vi "sub_Test_main.vi"(8 "error in":errorcluster) -> (0 "error out":errorcluster)   [LabVIEW 2019]
uses:
  _ctrl/create-rw-close.ctl
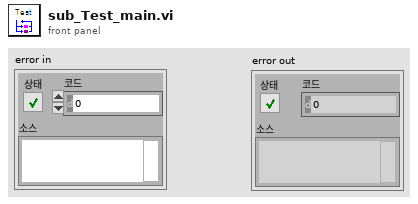
[diagram p1: front panel]
types:
  T1 = typedef "create-rw-close.ctl" = enum16{"create", "write", "read", "delete", "close"}
  T2 = typedef "fgv_Main_q.ctl" = enum16{"init", "wait", "R", "RC", "RC_M", "B1", "B2", "B3", "exit"}
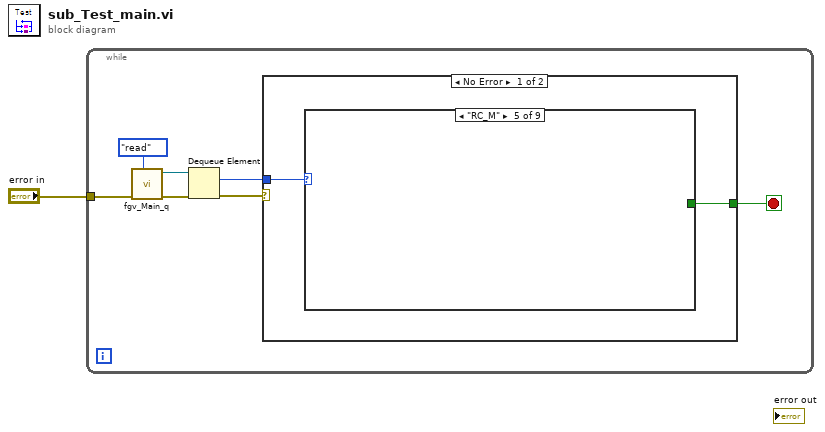
[diagram p0: block diagram]
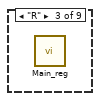
[diagram p4: hidden frame]
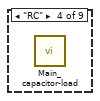
[diagram p5: hidden frame]
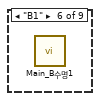
[diagram p6: hidden frame]
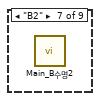
[diagram p7: hidden frame]
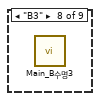
[diagram p8: hidden frame]
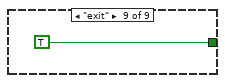
[diagram p9: hidden frame]
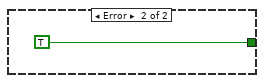
[diagram p10: hidden frame]
diagram:
  n1 = while {
    tunnel: "error in" -> [w2]
    stop <- w8 stop-if-true
    n2 = call "fgv_Main_q.vi"("cmd"=create-rw-close."read", "error in"=w2) -> ("error out"=w5:errorcluster, "queue out"=w6:refnum<queue>)  [unwired: 8 in]
    n3 = Dequeue Element(queue=w6, error in (no error)=w5) -> (element=w4:T2, error out=w3:errorcluster)  [unwired: 1 in, 2 out]
    n4 = case shown="No Error" w3 {
      tunnel: [w9 TRUE] -> w8
      tunnel: w4 -> [w10 _]
      frame No Error {
        n5 = case shown="\"RC_M\"" w10 {
          tunnel: [_ _ _ _ _ _ _ _ TRUE] -> w9
          frame "init", Default {
          }
          frame "wait" {
          }
          frame "R" {
            n6 = call "Main_reg.vi"() -> ()  [unwired: 12 in]
          }
          frame "RC" {
            n7 = call "Main_capacitor-load.vi"() -> ()  [unwired: 11 in, 1 out]
          }
          frame "RC_M" {
          }
          frame "B1" {
            n8 = call "Main_B수명1.vi"() -> ()  [unwired: 11 in, 1 out]
          }
          frame "B2" {
            n9 = call "Main_B수명2.vi"() -> ()  [unwired: 11 in, 1 out]
          }
          frame "B3" {
            n10 = call "Main_B수명3.vi"() -> ()  [unwired: 11 in, 1 out]
          }
          frame "exit" {
          }
        }
      }
      frame Error {
      }
    }
  }
